vi "BigAccDAQ.vi"() -> ()   [LabVIEW 2013]
uses:
  <vilib>/Utility/miscctls.llb/LVPointTypeDef.ctl
  <instrlib>/niScope/Controls/niScope vertical coupling.ctl
  <instrlib>/niScope/Controls/niScope trigger coupling.ctl
  <instrlib>/niScope/Controls/niScope trigger slope.ctl
  <instrlib>/niScope/Controls/niScope trigger source.ctl
  Controls/Dust_Event.ctl
  Controls/Signal.ctl
  Controls/Role ID.ctl
  Controls/Hardware ID.ctl
  Controls/Estimate_source.ctl
  <instrlib>/niScope/Configure/Trigger/niScope Configure Trigger Edge.vi
  <instrlib>/niScope/Acquire/Fetch/niScope Multi Fetch Cluster.vi
  Global Variables/PSU updated.vi
panel:
  in  "Filter":bool
  in  "Filter Half\nWidth":i32=10
  out "Detectors 1 and 2":waveform(dbl)[](graph)
  in  "Write to Database?":bool
  out "PSU":dynamicdata(graph)
  out "Detector 3":dynamicdata(graph)
  out "Avg. Rate":dbl format="%#.3g"
  in  "Ref. Pos.":dbl=40.0 format="%#_13g"
  in  "Reset Count":bool
  in  "min sample rate":dbl=1000000.0 format="%.2p"
  in  "Clear Errors?":bool
  out "No. of Events":i32
  out "error out":errorcluster
  in  "stop":bool
  in  "trigger level":dbl=0.5 format="%.4f"
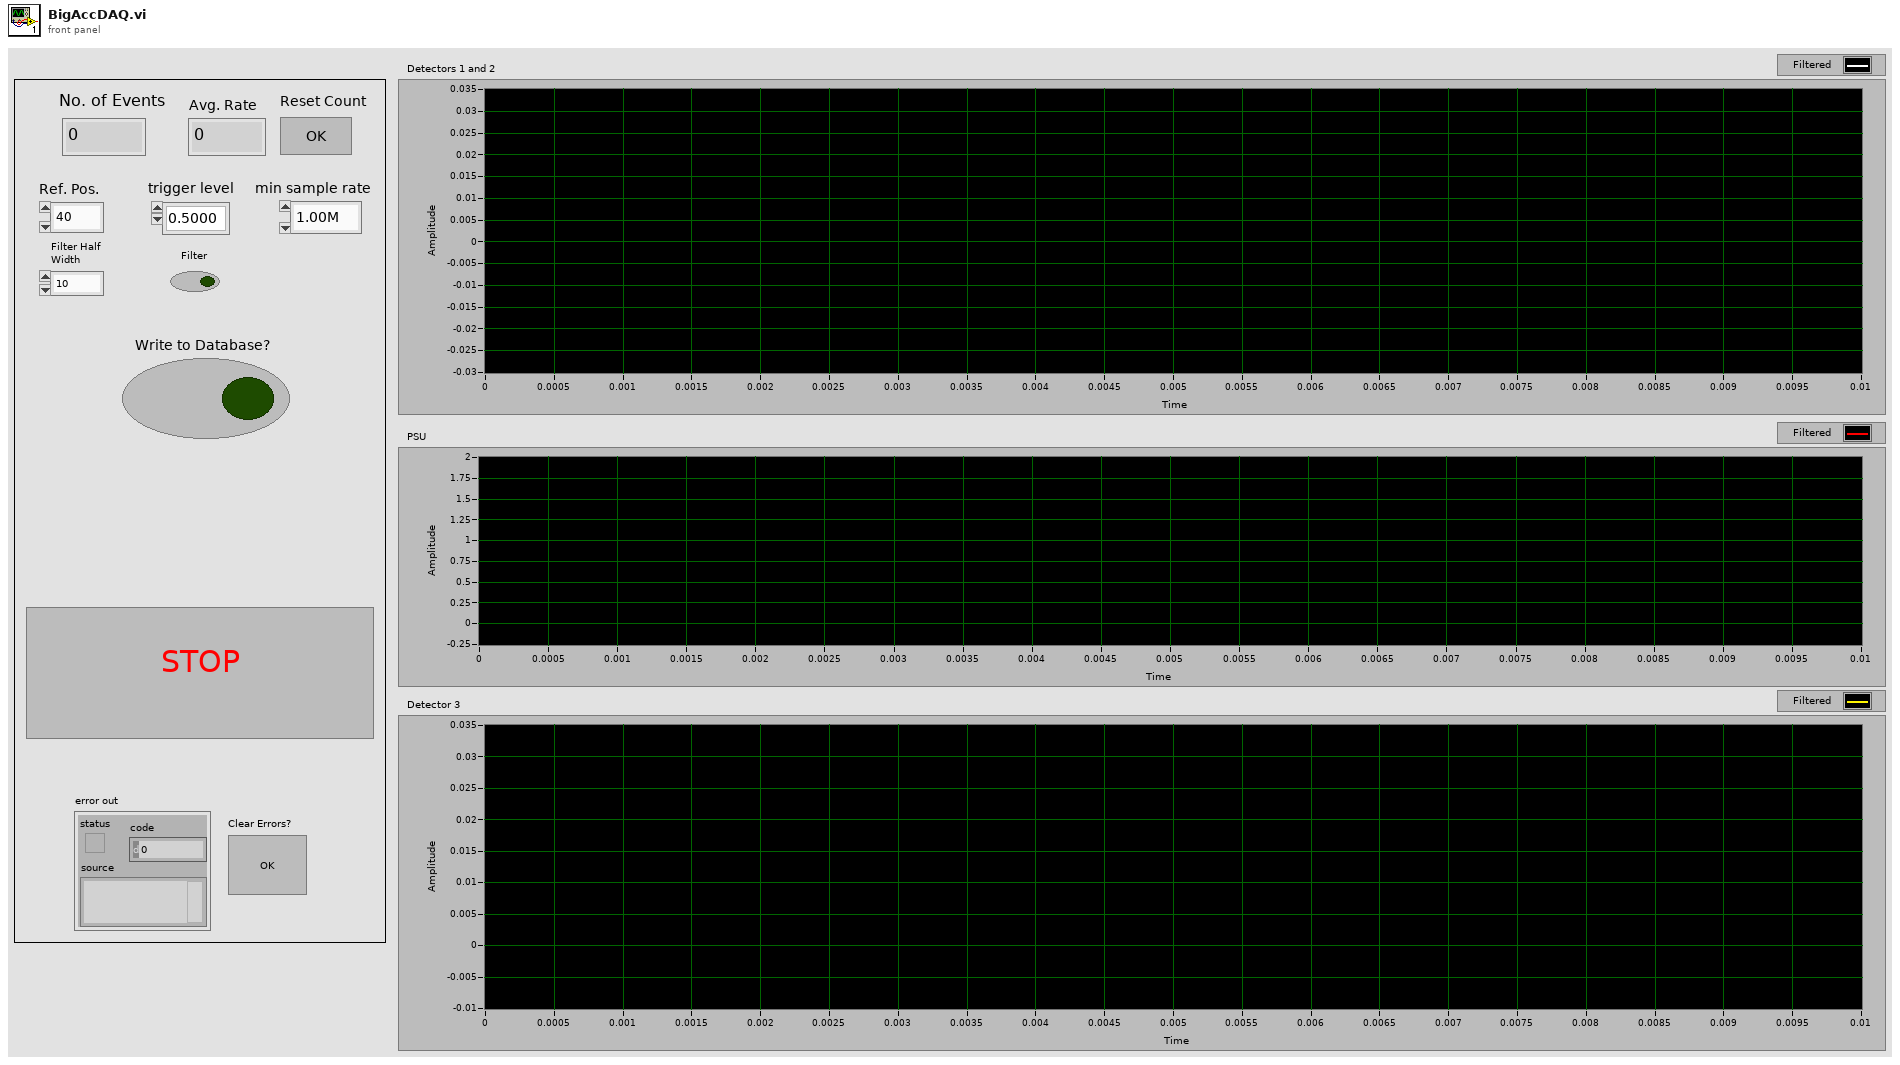
[diagram p1: front panel]
types:
  T1 = typedef "LVPointTypeDef.ctl" = cluster{"Horizontal":i16, "Vertical":i16}
  T2 = typedef "niScope trigger source.ctl" = string
  T3 = cluster{"relativeInitialX":dbl, "xIncrement":dbl, "wfm":dbl[]}[]
  T4 = typedef "Dust_Event.ctl" = cluster{"Time Stamp":timestamp, "Velocity":sgl, "Mass":sgl, "Charge":sgl, "Radius":sgl, "Array":T5[], "Dust Event ID":i64, "Passed_3rd_Detector":bool, "Estimate Source":T8, "Estimate Quality":sgl}
  T5 = typedef "Signal.ctl" = cluster{"Signal ID":i64, "Time Stamp":timestamp, "Dust Event ID":i64, "Role ID":T6, "Data":sgl[], "Signal Length":i32, "dt":sgl, "Offset":dbl, "Hardware ID":T7}
  T6 = typedef "Role ID.ctl" = enum16{"First_Detector", "Second_Detector", "Third_Detector", "LeCroy_CH1", "LeCroy_CH2", "LeCroy_CH3", "LeCroy_CH4", "PSU", "DCS 1", "DCS 2"}
  T7 = typedef "Hardware ID.ctl" = enum16{"Unknown", "CSA 1", "CSA 2", "CSA 3", "CSA 4", "CSA 5", "CSA 6", "DCS 1", "DCS 2"}
  T8 = typedef "Estimate_source.ctl" = i8
  T9 = typedef "niScope vertical coupling.ctl" = i32
  T10 = typedef "niScope trigger slope.ctl" = i32
  T11 = typedef "niScope trigger coupling.ctl" = u16
  T12 = cluster{"relativeInitialX":dbl, "xIncrement":dbl, "wfm":dbl[]}
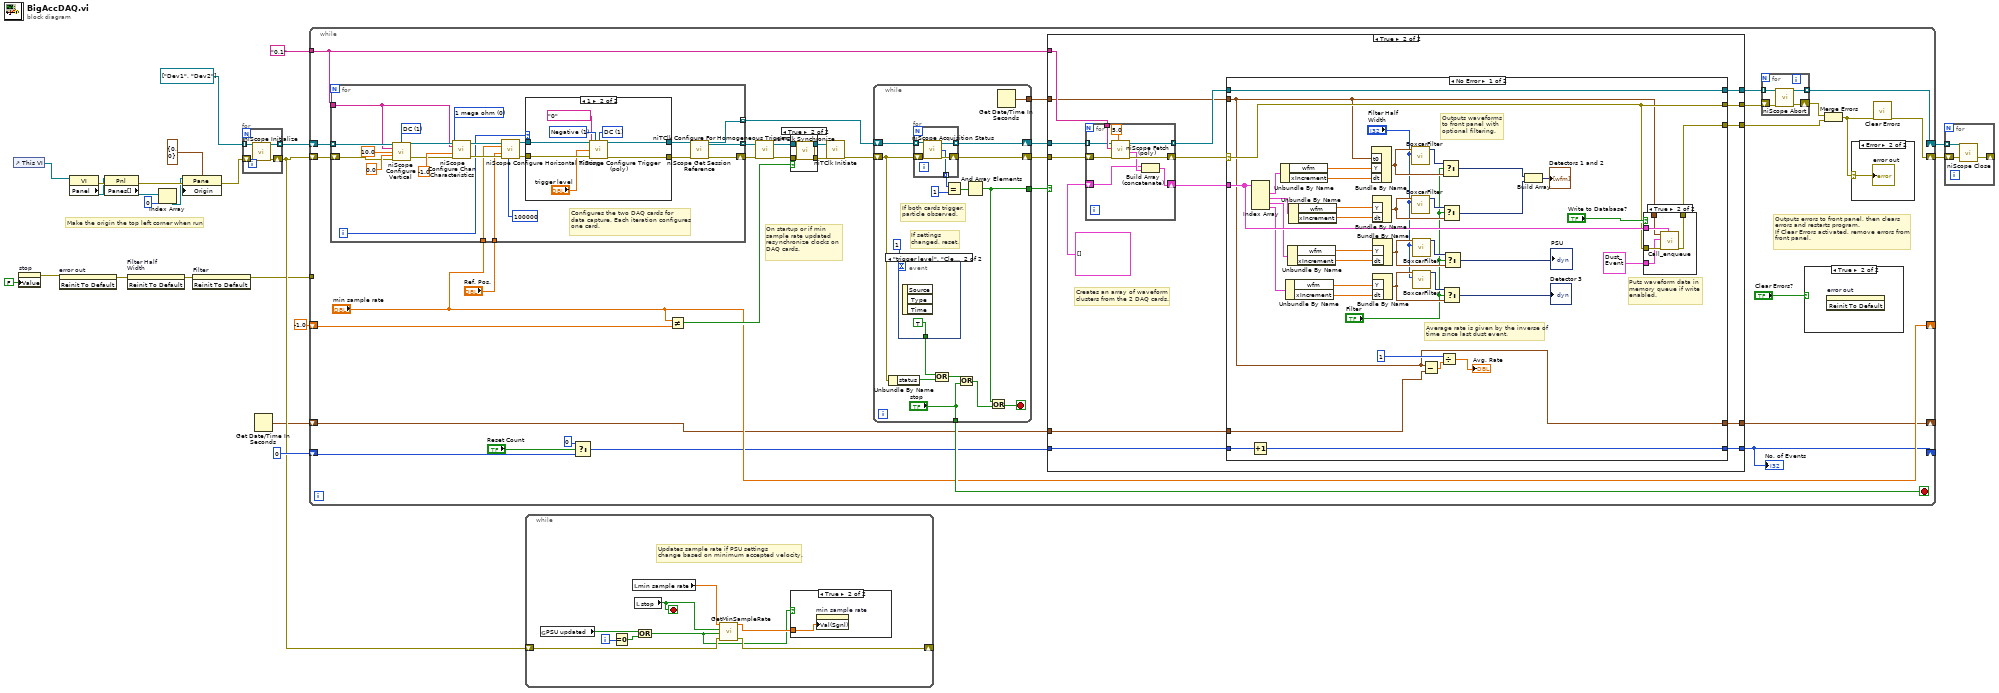
[diagram p0: block diagram]
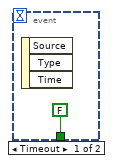
[diagram p8: hidden frame]
diagram:
  # "Make the origin the top left corner when run"
  n1 = control-ref of="This VI"() -> (w15:refnum<vi>)
  n2 = property on="stop" class="Bool (strict)"("Value"=FALSE ("stop")) -> (error out=w7:errorcluster)  [unwired: 2 in, 1 out]
  n3 = invoke on="error out" class="Clust (strict)" method="Reinit To Default"(error in=w7) -> (error out=w3:errorcluster)  [unwired: 2 in, 2 out]
  n4 = property class="VI"(reference=w15) -> (error out=w22:errorcluster, "Panel"=w16:refnum<vi>)  [unwired: 1 in, 1 out]
  n5 = property class="Pnl"(reference=w16, error in=w22) -> (error out=w21:errorcluster, "Panes[]"=w20:refnum<vi>[])  [unwired: 1 out]
  n6 = invoke on="Filter Half\nWidth" class="DigNum (strict)" method="Reinit To Default"(error in=w3) -> (error out=w2:errorcluster)  [unwired: 2 in, 2 out]
  n7 = Index Array(array=w20, index=0) -> (element=w18:refnum<vi>)
  n8 = property class="Pane"(reference=w18, error in=w21, "Origin"=T1 {"Horizontal"=0, "Vertical"=0}) -> (error out=w23:errorcluster)  [unwired: 1 out]
  n9 = invoke on="Filter" class="Bool (strict)" method="Reinit To Default"(error in=w2) -> (error out=w1:errorcluster)  [unwired: 2 in, 2 out]
  n10 = for {
    tunnel: [w25] -> w12 mode=indexing
    tunnel: refnum<k15>[] ["Dev1", "Dev2"] -> [w24] mode=indexing
    shift-right: [w26] -> w9
    shift-left: w23 -> [w27]
    n11 = call <instrlib>:"niScope Initialize.vi"("resource name"=w24, "error in"=w27) -> ("instrument handle"=w25:refnum<k15>, "error out"=w26:errorcluster)  [unwired: 12 in]
  }
  n12 = Get Date/Time In Seconds() -> (seconds since 1Jan1904=w6:timestamp)
  n13 = while {
    tunnel: "0,1" ("channels") -> [w39]
    shift-right: [w49] -> w5
    shift-left: w12 -> [w61]
    shift-right: [w48] -> w4
    shift-left: w9 -> [w62]
    shift-right: [w30] -> _
    shift-left: 0 -> [w33]
    shift-right: ["min sample rate"] -> _
    shift-left: -1.0 ("min sample rate") -> [w44]
    shift-right: [w35] -> _
    shift-left: w6 -> [w37]
    tunnel: w1 -> [_]
    stop <- w45 stop-if-true
    # "Outputs errors to front panel, then clears \nerrors and restarts program. \nIf Clear Errors activated, remove errors from \nfront panel."
    # "On startup or if min \nsample rate updated\nresynchronize clocks on \nDAQ cards."
    n14 = for {
      tunnel: w61 -> [w91] mode=indexing
      tunnel: [w78] -> w43 mode=indexing
      tunnel: w39 -> [w80]
      shift-right: [w76] -> w54
      shift-left: w62 -> [w92]
      tunnel: [w75] -> w55 mode=indexing
      tunnel: "min sample rate" -> [w73]
      tunnel: "Ref. Pos." -> [w74]
      i -> [w79]
      w90 = u32 0 items=["1 mega ohm"=0, "50 ohms"=2] ("input impedance")
      w93 = T9 1 items=["AC", "DC", "Ground"] ("vertical coupling")
      # "Configures the two DAQ cards for \ndata capture. Each iteration configures\none card."
      n15 = call <instrlib>:"niScope Configure Vertical.vi"("instrument handle"=w91, "vertical coupling"=w93, "channels"=w80, "vertical range"=10.0, "vertical offset"=0.0, "error in"=w92) -> ("instrument handle out"=w87:refnum<k15>, "error out"=w88:errorcluster)  [unwired: 8 in]
      n16 = call <instrlib>:"niScope Configure Chan Characteristics.vi"("instrument handle"=w87, "channels"=w80, "input impedance"=w90, "maximum input frequency"=-1.0, "error in"=w88) -> ("instrument handle out"=w84:refnum<k15>, "error out"=w85:errorcluster)  [unwired: 9 in]
      n17 = call <instrlib>:"niScope Configure Horizontal Timing.vi"("instrument handle"=w84, "min sample rate"=w73, "reference position"=w74, "error in"=w85, "min record length"=100000) -> ("instrument handle out"=w83:refnum<k15>, "error out"=w82:errorcluster)  [unwired: 9 in]
      n18 = case shown="1" w79 {
        tunnel: w83 -> [w97 w105]
        tunnel: w82 -> [w96 w104]
        tunnel: [w97 w99] -> w81
        tunnel: [w96 w98] -> w77
        frame 0, Default {
        }
        frame 1 {
          w102 = T10 1 items=["Positive", "Negative"] ("trigger slope")
          w103 = T11 1 items=["AC"=0, "DC"=1, "HF Reject"=3, "LF Reject"=4, "AC Plus HF Reject"=1001] ("trigger coupling")
          n19 = call-poly <instrlib>:"niScope Configure Trigger (poly).vi"("instrument handle"=w105, "trigger slope"=w102, "trigger coupling"=w103, "trigger source"=T2 "0", "trigger level"="trigger level", "error in"=w104) -> ("instrument handle out"=w99:refnum<k15>, "error out"=w98:errorcluster)  [unwired: 8 in]
        }
      }
      n20 = call <instrlib>:"niScope Get Session Reference.vi"("instrument handle"=w81, "error in"=w77) -> ("instrument handle out"=w78:refnum<k15>, "session reference"=w75:refnum<k20>, "error out"=w76:errorcluster)  [unwired: 11 in]
    }
    n21 = Select(t=0, s="Reset Count", f=w33) -> (s? t:f=w36:i32)
    n22 = Not Equal?(x="min sample rate", y=w44) -> (x != y?=w47:bool)
    n23 = call <instrlib>:"niTClk Configure For Homogeneous Triggers.vi"("error in (no error)"=w54, "sessions"=w55) -> ("error out"=w52:errorcluster, "sessions out"=w53:refnum<k20>[])  [unwired: 8 in]
    n24 = case shown="True" w47 {
      tunnel: w53 -> [w64 w68]
      tunnel: w52 -> [w63 w67]
      tunnel: [w64 w66] -> w51
      tunnel: [w63 w65] -> w50
      frame False {
      }
      frame True {
        n25 = call <instrlib>:"niTClk Synchronize.vi"("error in (no error)"=w67, "sessions"=w68) -> ("error out"=w65:errorcluster, "sessions out"=w66:refnum<k20>[])  [unwired: 8 in]
      }
    }
    n26 = call <instrlib>:"niTClk Initiate.vi"("error in (no error)"=w50, "sessions"=w51) -> ("error out"=w34:errorcluster)  [unwired: 8 in, 1 out]
    n27 = while {
      shift-right: [w198] -> w58
      shift-left: w43 -> [w199]
      shift-right: [w190] -> w57
      shift-left: w34 -> [w187]
      tunnel: [w186] -> w56
      tunnel: [w192] -> w38
      tunnel: ["stop"] -> w45
      stop <- w189 stop-if-true
      # "If settings \nchanged, reset."
      # "If both cards trigger,\nparticle observed."
      n28 = Unbundle By Name(w187) -> ("status"=w184:bool)
      n29 = event shown="[1] \"trigger level\", \"Clear Errors?\", \"min sample rate\", \"Reset Count\", \"Ref. Pos.\": Value Change" {
        selector: _ -> [_ _]
        dyn-events: _ -> [_ _]
        timeout: 1 -> [_ _]
        tunnel: [FALSE TRUE] -> w185
        event Timeout {
          n30 = event-data() -> ()  [unwired: 1 in, 3 out]
        }
        event "trigger level", "Clear Errors?", "min sample rate", "Reset Count", "Ref. Pos.": Value Change {
          n31 = event-data() -> ()  [unwired: 1 in, 3 out]
        }
      }
      n32 = for {
        tunnel: w199 -> [w204] mode=indexing
        tunnel: [w201] -> w198 mode=indexing
        tunnel: [w200] -> w197 mode=indexing
        shift-right: [w202] -> w190
        shift-left: w187 -> [w203]
        n33 = call <instrlib>:"niScope Acquisition Status.vi"("instrument handle"=w204, "error in"=w203) -> ("instrument handle out"=w201:refnum<k15>, "acquisition status"=w200:i32, "error out"=w202:errorcluster)  [unwired: 11 in]
      }
      n34 = Or(x=w185, y=w184) -> (x .or. y?=w194:bool)
      n35 = Equal?(x=w197, y=1) -> (x = y?=w193:bool[])
      n36 = Or(x=w194, y="stop") -> (x .or. y?=w188:bool)
      n37 = And Array Elements(Boolean array=w193) -> (logical AND=w186:bool)
      n38 = Or(x=w186, y=w188) -> (x .or. y?=w189:bool)
      n39 = Get Date/Time In Seconds() -> (seconds since 1Jan1904=w192:timestamp)
    }
    n40 = case shown="True" w56 {
      tunnel: [w109 w113] -> w31
      tunnel: [w106 w111] -> w28
      tunnel: w58 -> [w109 w124]
      tunnel: w57 -> [w106 w123]
      tunnel: [w106 w112] -> w32
      tunnel: w39 -> [_ w118]
      tunnel: w38 -> [_ w117]
      tunnel: w37 -> [w107 w116]
      tunnel: w36 -> [w108 w115]
      tunnel: [w108 w114] -> w30
      tunnel: [w107 w110] -> w35
      frame False {
      }
      frame True {
        # "Creates an array of waveform \nclusters from the 2 DAQ cards."
        n41 = for {
          tunnel: w118 -> [w183]
          tunnel: [w181] -> w120 mode=indexing
          tunnel: w124 -> [w179] mode=indexing
          shift-right: [w176] -> w119
          shift-left: T3 [] ("waveform") -> [w175]
          shift-right: [w180] -> w121
          shift-left: w123 -> [w178]
          n42 = call-poly <instrlib>:"niScope Fetch (poly).vi"("timeout"=5.0, "error in"=w178, "channels"=w183, "instrument handle"=w179) -> ("error out"=w180:errorcluster, "waveform"=w177:T3, "instrument handle out"=w181:refnum<k15>)  [unwired: 4 in, 1 out]
          n43 = Build Array (concatenate)(w175, w177) -> (w176:T3)
        }
        n44 = case shown="No Error" w121 {
          selector: w121 -> [w157 w174]
          tunnel: w119 -> [w161 _]
          tunnel: w120 -> [w159 w173]
          tunnel: [w159 w173] -> w113
          tunnel: [w160 w174] -> w111
          tunnel: w115 -> [w158 w172]
          tunnel: [w154 w172] -> w114
          tunnel: [w157 w174] -> w112
          tunnel: w117 -> [w152 _]
          tunnel: w116 -> [w143 w171]
          tunnel: [w152 w171] -> w110
          frame No Error {
            # "Puts waveform data in\nmemory queue if write \nenabled."
            # "Outputs waveforms\nto front panel with\noptional filtering."
            # "Average rate is given by the inverse of \ntime since last dust event."
            n45 = Increment(x=w158) -> (x+1=w154:i32)
            n46 = Index Array(array=w161) -> (element #1=w164:T12, element #2=w163:T12, element #3=w156:T12, element #4=w155:T12)  [unwired: 4 in]
            n47 = Unbundle By Name(w164) -> ("wfm"=w151:dbl[], "xIncrement"=w150:dbl)
            n48 = Unbundle By Name(w155) -> ("wfm"=w146:dbl[], "xIncrement"=w145:dbl)
            n49 = Unbundle By Name(w156) -> ("wfm"=w147:dbl[], "xIncrement"=w144:dbl)
            n50 = Unbundle By Name(w163) -> ("wfm"=w149:dbl[], "xIncrement"=w148:dbl)
            n51 = Bundle By Name("t0"=w152, "Y"=w151, "dt"=w150) -> (w131:waveform(dbl))  [unwired: 1 in]
            n52 = Bundle By Name("Y"=w149, "dt"=w148) -> (w133:waveform(dbl))  [unwired: 1 in]
            n53 = Bundle By Name("Y"=w147, "dt"=w144) -> (w136:waveform(dbl))  [unwired: 1 in]
            n54 = Bundle By Name("Y"=w146, "dt"=w145) -> (w139:waveform(dbl))  [unwired: 1 in]
            n55 = call "BoxcarFilter.vi"("Half Width"="Filter Half\nWidth", "Signal"=w131) -> ("Filtered Signal"=w129:dynamicdata)  [unwired: 8 in, 1 out]
            n56 = call "BoxcarFilter.vi"("Half Width"="Filter Half\nWidth", "Signal"=w133) -> ("Filtered Signal"=w132:dynamicdata)  [unwired: 8 in, 1 out]
            n57 = call "BoxcarFilter.vi"("Half Width"="Filter Half\nWidth", "Signal"=w136) -> ("Filtered Signal"=w135:dynamicdata)  [unwired: 8 in, 1 out]
            n58 = call "BoxcarFilter.vi"("Half Width"="Filter Half\nWidth", "Signal"=w139) -> ("Filtered Signal"=w138:dynamicdata)  [unwired: 8 in, 1 out]
            n59 = Subtract(x=w152, y=w143) -> (x-y=w141:dbl)
            n60 = Divide(x=1 ("y"), y=w141) -> (x/y=→"Avg. Rate":dbl)
            n61 = Select(t=w129, s="Filter", f=w131) -> (s? t:f=w128:dynamicdata)
            n62 = Select(t=w132, s="Filter", f=w133) -> (s? t:f=w127:dynamicdata)
            n63 = Select(t=w138, s="Filter", f=w139) -> (s? t:f=→"Detector 3":dynamicdata)
            n64 = Select(t=w135, s="Filter", f=w136) -> (s? t:f=→"PSU":dynamicdata)
            n65 = Build Array(w128, w127) -> (→"Detectors 1 and 2":dynamicdata[])
            n66 = case shown="True" "Write to Database?" {
              tunnel: w161 -> [_ w170]
              tunnel: w157 -> [w165 w169]
              tunnel: [w165 w168] -> w160
              tunnel: w152 -> [_ w167]
              tunnel: T4 {"Time Stamp"=timestamp(0 s since 1904-01-01), "Velocity"=0.0, "Mass"=0.0, "Charge"=0.0, "Radius"=0.0, "Array"=[], "Dust Event ID"=0, "Passed_3rd_Detector"=FALSE, "Estimate Source"=0, "Estimate Quality"=0.0} ("Input Data") -> [_ w166]
              frame False {
              }
              frame True {
                n67 = call "Call_enqueue.vi"("Waveform"=w170, "error in"=w169, "Input Data"=w166, "Timestamp"=w167) -> ("error out"=w168:errorcluster)  [unwired: 7 in]
              }
            }
          }
          frame Error {
          }
        }
      }
    }
    "No. of Events" <- w30
    n68 = for {
      shift-right: [w72] -> w29
      shift-left: w32 -> [w71]
      tunnel: [w70] -> w49 mode=indexing
      tunnel: w31 -> [w69] mode=indexing
      n69 = call <instrlib>:"niScope Abort.vi"("instrument handle"=w69, "error in"=w71) -> ("instrument handle out"=w70:refnum<k15>, "error out"=w72:errorcluster)  [unwired: 12 in]
    }
    n70 = case shown="True" "Clear Errors?" {
      frame False {
      }
      frame True {
        n71 = invoke on="error out" class="Clust (strict)" method="Reinit To Default"() -> ()  [unwired: 3 in, 3 out]
      }
    }
    n72 = Merge Errors(w29, w28) -> (w60:errorcluster)
    n73 = case shown="Error" w60 {
      selector: w60 -> [_ w207]
      frame No Error {
      }
      frame Error {
        "error out" <- w207
      }
    }
    n74 = call <vilib>:"Clear Errors.vi"("error in (no error)"=w60) -> ("error out"=w48:errorcluster)  [unwired: 6 in]
  }
  n75 = while {
    shift-right: [w210] -> _
    shift-left: w9 -> [w213]
    i -> [w216]
    stop <- w212 stop-if-true
    # "Updates sample rate if PSU settings \nchange based on minimum accepted velocity."
    n76 = global read "PSU updated.vi" "PSU updated"() -> (w215:bool)
    n77 = Equal To 0?(x=w216) -> (x = 0?=w214:bool)
    n78 = local read "min sample rate"() -> (w211:dbl)
    n79 = local read "stop"() -> (w212:bool)
    n80 = Or(x=w215, y=w214) -> (x .or. y?=w208:bool)
    n81 = call "GetMinSampleRate.vi"("error in (no error)"=w213, "PSU Update"=w208, "stop"=w212, "min sample rate"=w211) -> ("error out"=w210:errorcluster, "min sample rate"=w209:dbl)  [unwired: 6 in]
    n82 = case shown="True" w208 {
      tunnel: w209 -> [_ w217]
      frame False {
      }
      frame True {
        n83 = property on="min sample rate" class="DigNum (strict)"("Val(Sgnl)"=w217) -> ()  [unwired: 2 in, 2 out]
      }
    }
  }
  n84 = for {
    tunnel: w5 -> [w220] mode=indexing
    shift-right: [w218] -> _
    shift-left: w4 -> [w219]
    n85 = call <instrlib>:"niScope Close.vi"("instrument handle"=w220, "error in"=w219) -> ("error out"=w218:errorcluster)  [unwired: 13 in]
  }
